vi "PH_PowerUnit_BaseClass.contents.vi"   [LabVIEW 2014, in "PH_PowerUnit_BaseClass.lvlib"]
doc: "This class is forseen to control a PreAmp Power Unit. Actually it controls several device layer classes. The head itself is fully operational, but should be used via the PHELIX_Sequencer class only. It has an own state machine.\n\nThis class is part of the PHELIX application layer."
uses:
  PH_PowerUnit_BaseClass.lvlib
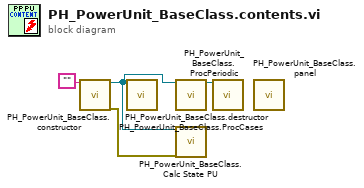
[diagram p0: block diagram]
diagram:
  n1 = call "PH_PowerUnit_BaseClass.constructor.vi"("name"="") -> ("i ref out"=w2:refnum<vi>, "error out"=w1:errorcluster)  [unwired: 16 in, 1 out]
  n2 = call "PH_PowerUnit_BaseClass.destructor.vi"("i ref in"=w2) -> ()  [unwired: 18 in, 1 out]
  n3 = call "PH_PowerUnit_BaseClass.ProcCases.vi"("i ref in"=w2) -> ("i ref out"=w4:refnum<vi>)  [unwired: 16 in, 2 out]
  n4 = call "PH_PowerUnit_BaseClass.Calc State PU.vi"("i ref in"=w2, "error in (no error)"=w1) -> ()  [unwired: 16 in, 2 out]
  n5 = call "PH_PowerUnit_BaseClass.ProcPeriodic.vi"("i ref in"=w4) -> ()  [unwired: 16 in, 3 out]
  n6 = call "PH_PowerUnit_BaseClass.panel.vi"() -> ()  [unwired: 1 in]
